vi "Clear Cache.vi"   [LabVIEW 2016]
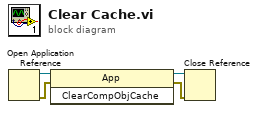
[diagram p0: block diagram]
diagram:
  n1 = Open Application Reference() -> (0:w1:errorcluster, 3:w4:refnum<vi>)  [unwired: 4 in]
  n2 = invoke class="App" method="ClearCompObjCache"(reference=w4, error in=w1) -> (reference out=w3:refnum<vi>, error out=w2:errorcluster)  [unwired: 1 in, 1 out]
  n3 = Close Reference(reference=w3, error in (no error)=w2) -> ()  [unwired: 1 out]
